vi "Generate Simulated Data.vi"(8 "error in (no error)":errorcluster) -> (0 "error out":errorcluster, 2 "Numeric":dbl)   [LabVIEW 2023, in "Acquisition.lvlib"]
doc: "Generates sample waveforms according to the signal type in the HW Config input."
uses:
  Acquisition.lvlib
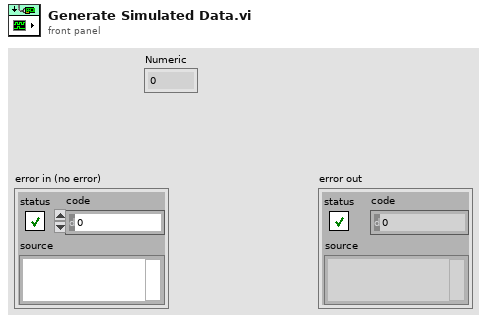
[diagram p1: front panel]
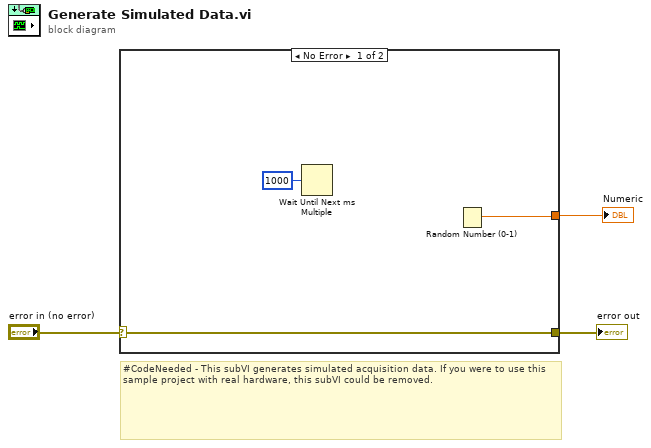
[diagram p0: block diagram]
diagram:
  # "#CodeNeeded - This subVI generates simulated acquisition data. If you were to use this sample project with real hardware, this subVI could be removed."
  n1 = case shown="No Error" "error in (no error)" {
    selector: "error in (no error)" -> [w6 w7]
    tunnel: [w6 w7] -> w2
    tunnel: [w4 _] -> w1
    frame No Error {
      n2 = Wait Until Next ms Multiple(millisecond multiple=u32 1000) -> ()  [unwired: 1 out]
      n3 = Random Number (0-1)() -> (number: 0 to 1=w4:dbl)
    }
    frame Error {
    }
  }
  "error out" <- w2
  "Numeric" <- w1
